vi "Stream Split Character Match RegExp Std Out.vi"(8 "error in (no error)":errorcluster, 11 "configuration in":refnum<class "configuration.lvclass">) -> (0 "error out":errorcluster, 2 "Stream Split Character Match RegExp Std Out":string)   [LabVIEW 2024, in "serenial.io-ase.lvlib" / "configuration.lvclass"]
doc: "Specify the regular expression that will be used to match the breaks in the Standard Output stream.\n\nThis library uses the PERL regexp library syntax."
uses:
  configuration/configuration.lvclass
  configuration/configuration.lvclass/configuration.ctl
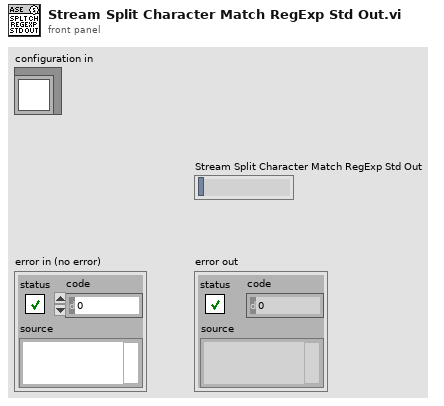
[diagram p1: front panel]
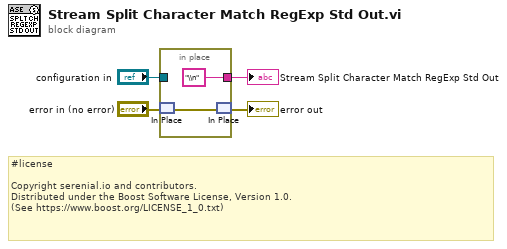
[diagram p0: block diagram]
diagram:
  # "#license\n\nCopyright serenial.io and contributors.\nDistributed under the Boost Software License, Version 1.0.\n(See https://www.boost.org/LICENSE_1_0.txt)"
  n1 = in-place "In Place Element Structure" {
    in-place-border: "configuration in" -> [_]
    in-place-border: ["\\n"] -> w1
    n2 = in-place-match #1 ("In Place In / Out Element")("error in (no error)") -> (w6:errorcluster)
    n3 = in-place-match #1 ("In Place In / Out Element")(w6) -> (→"error out":errorcluster)
  }
  "Stream Split Character Match RegExp Std Out" <- w1
